vi "is AH bridge.vi"(8 "Error In":errorcluster, 11 "VISA resource name":refnum<visa-resource-name>) -> (0 "Error Out":errorcluster, 2 "Is AH?":bool, 3 "VISA resource name out":refnum<visa-resource-name>)   [LabVIEW 2021]
uses:
  GPIB/VISA  Send Receive.vi
  Simple VISA Reader/Simple VISA Reader Driver.lvclass
panel:
  out "data string out":string
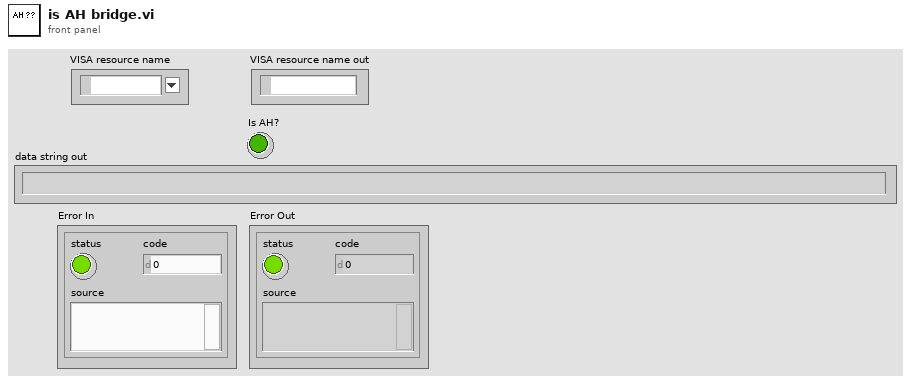
[diagram p1: front panel]
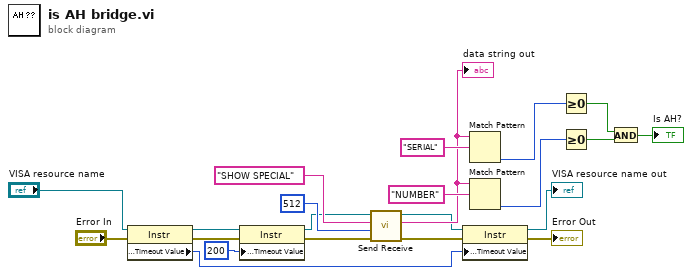
[diagram p0: block diagram]
diagram:
  n1 = property class="Instr"(reference="VISA resource name", error in="Error In") -> (reference out=w13:refnum<visa-resource-name>, error out=w12:errorcluster, "General Settings:Timeout Value"=w6:u32)
  n2 = property class="Instr"(reference=w13, error in=w12, "General Settings:Timeout Value"=u32 200) -> (reference out=w9:refnum<visa-resource-name>, error out=w10:errorcluster)
  n3 = call-poly "Send Receive.vi"("error in (no error)"=w10, "Receive count"=512 ("read count"), "data string in"="SHOW SPECIAL" ("write buffer"), "VISA Resource Name"=w9) -> ("error out"=w8:errorcluster, "data string out"=w16:string, "VISA Resource Name Out"=w7:refnum<visa-resource-name>)  [unwired: 5 in]
  "data string out" <- w16
  n4 = property class="Instr"(reference=w7, error in=w8, "General Settings:Timeout Value"=w6) -> (reference out=→"VISA resource name out":refnum<visa-resource-name>, error out=→"Error Out":errorcluster)
  n5 = Match Pattern(string=w16, regular expression="SERIAL") -> (offset past match=w20:i32)  [unwired: 4 out]
  n6 = Match Pattern(string=w16, regular expression="NUMBER") -> (offset past match=w17:i32)  [unwired: 4 out]
  n7 = Greater Or Equal To 0?(x=w20) -> (x >= 0?=w19:bool)
  n8 = Greater Or Equal To 0?(x=w17) -> (x >= 0?=w15:bool)
  n9 = And(x=w19, y=w15) -> (x .and. y?=→"Is AH?":bool)
